vi "Read Power Sensor.vi"(8 "error in (no error)":errorcluster, 10 "Instance (1)":i32=1 format="%.0g", 11 "VISA resource name":refnum<visa-resource-name>) -> (0 "error out":errorcluster, 1 "Power":dbl[](array[numeric]) format="%^.3e", 2 "Reliability":i32, 3 "VISA resource name out":refnum<visa-resource-name>, 4 "Elapsed Statistics":i32)   [LabVIEW 2020, in "Rohde&Schwarz CMXP GPRF.lvlib"]
doc: "Starts a new single shot measurement and returns the results.\n\nAttribute:\nRSCMXPGPRF_ATTR_READ_POWER_SENSOR\n\nRemote-control command:\nREAD:GPRF:MEAS<i>:EPSensor?"
uses:
  <instrlib>/Rohde&Schwarz CMXP GPRF/Rohde&Schwarz CMXP GPRF.lvlib
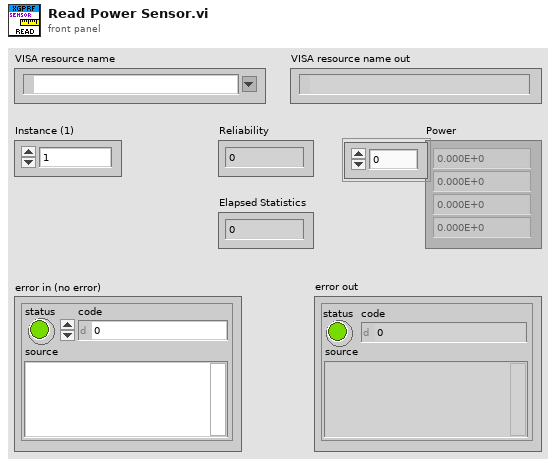
[diagram p1: front panel]
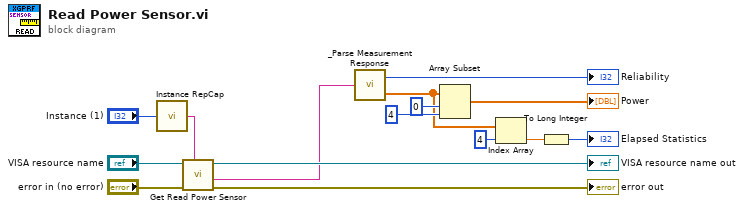
[diagram p0: block diagram]
diagram:
  n1 = call <instrlib>:"Instance RepCap.vi"("Instance in"="Instance (1)") -> ("Instance out"=w10:string)
  n2 = call "Get Read Power Sensor"("Repeated Capabilities"=w10, "error in (no error)"="error in (no error)", "instrument handle"="VISA resource name") -> ("error out"=→"error out":errorcluster, "Read Power Sensor"=w1:string, "instrument handle out"=→"VISA resource name out":refnum<visa-resource-name>)  [unwired: 6 in]
  n3 = call <instrlib>:"_Parse Measurement Response.vi"("String In"=w1) -> ("Reliability"=→"Reliability":i32, "Data"=w2:dbl[])
  n4 = Array Subset(array=w2, index=0, length=4) -> (→"Power":dbl[])
  n5 = Index Array(array=w2, index=4) -> (element=w5:dbl)
  n6 = To Long Integer(number=w5) -> (32bit integer=→"Elapsed Statistics":i32)
